vi "Img Plot Box.vi"(6 "Color":cluster{"Frame Color":u32, "Fill Color":u32}={"Frame Color"=16740207, "Fill Color"=16740207}, 8 "error in (no error)":errorcluster, 10 "Rectangle":T2, 11 "Image in":T1) -> (0 "error out":errorcluster, 3 "Image Out":T1)   [LabVIEW 2018, in "Image Process.lvclass"]
uses:
  Image Process.lvclass
  <vilib>/vision/Image Controls.llb/IMAQ Image.ctl
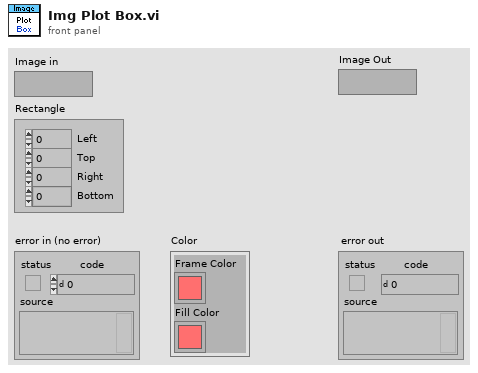
[diagram p1: front panel]
types:
  T1 = typedef "IMAQ Image.ctl" = refnum<image>
  T2 = cluster{"Left":i32, "Top":i32, "Right":i32, "Bottom":i32}
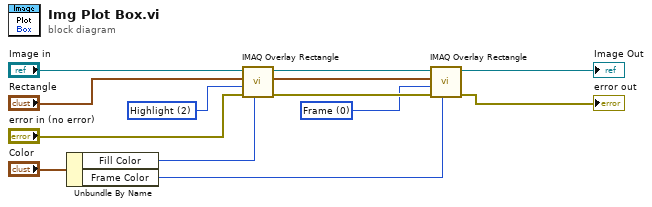
[diagram p0: block diagram]
diagram:
  w7 = u32 0 items=["Frame", "Fill", "Highlight"] ("Drawing Mode (Frame)")
  w12 = u32 2 items=["Frame", "Fill", "Highlight"] ("Drawing Mode (Frame)")
  n1 = Unbundle By Name("Color") -> ("Fill Color"=w5:u32, "Frame Color"=w4:u32)
  n2 = call "IMAQ Overlay Rectangle"("Color"=w5, "error in (no error)"="error in (no error)", "Drawing Mode (Frame)"=w12, "Rectangle"="Rectangle", "Image"="Image in") -> ("error out"=w8:errorcluster, "Image Out"=w9:T1)  [unwired: 5 in]
  n3 = call "IMAQ Overlay Rectangle"("Color"=w4, "error in (no error)"=w8, "Drawing Mode (Frame)"=w7, "Rectangle"="Rectangle", "Image"=w9) -> ("error out"=→"error out":errorcluster, "Image Out"=→"Image Out":T1)  [unwired: 5 in]
